vi "Update_Attribute_Tree_POLARIS.vi"(4 "Flush Tree?":bool, 5 "error in":errorcluster, 6 "Filter":string, 7 "Tree Control In":refnum<vi>, 8 "Camera Name In":T1 caption="Session In") -> (0 "error out":errorcluster, 2 "Tree Control Out":refnum<vi>, 3 "Session Out":T1)   [LabVIEW 2014, in "Camera Settings Dialog.lvlib" / "Camera Settings Dialog.lvclass"]
doc: "The Update Attribute Tree subVI, enumerates the attributes available for the camera and populates the Attribute Tree control with the attribute list."
uses:
  Camera Settings Dialog.lvclass
  <vilib>/userdefined/High Color/IMAQdx.ctl
  <vilib>/vision/driver/NI_Vision_Acquisition_Software.lvlib
  <resource>/objmgr/imaqdx.rc
panel:
  out "ValuesArray":string[](array[string])
  out "AttibuteArray":string[](array[string])
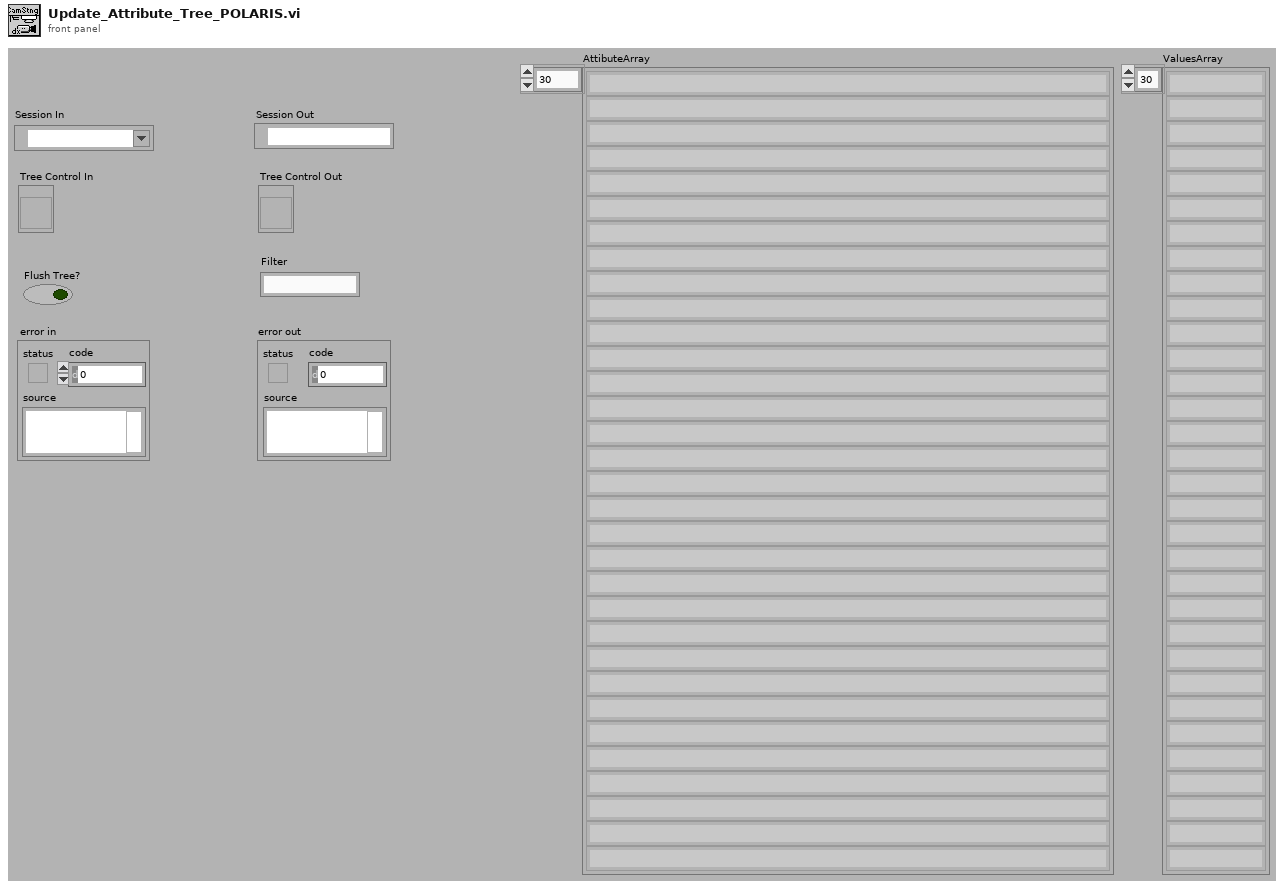
[diagram p1: front panel]
types:
  T1 = typedef "IMAQdx.ctl" = refnum<k21>
  T2 = typedef "NI_Vision_Acquisition_Software.lvlib/IMAQdx Attribute Type.ctl" = enum32{"U32", "I64", "DBL", "String", "Enum", "Bool", "Command"}
  T3 = cluster{"Attribute Type":T2, "Readable":bool, "Writable":bool, "Attribute Name":string}[]
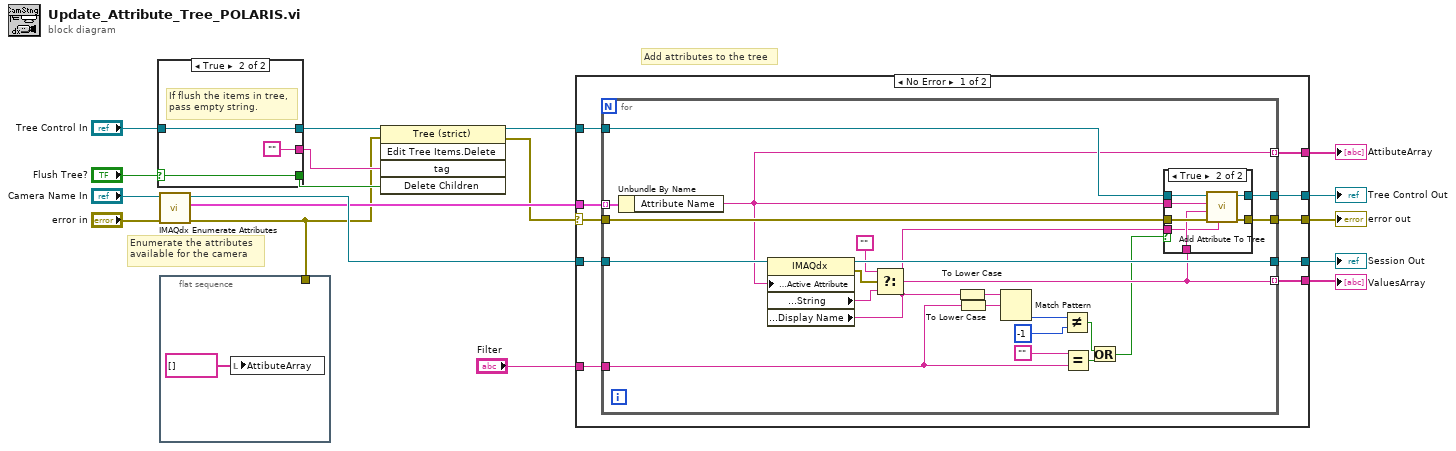
[diagram p0: block diagram]
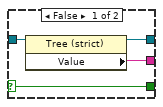
[diagram p2: hidden frame]
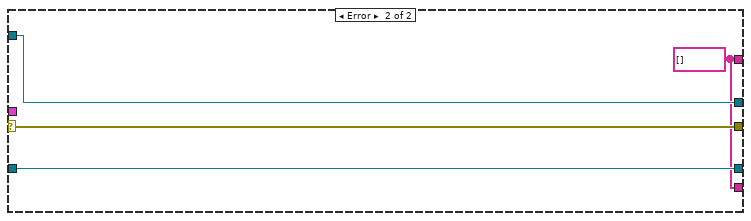
[diagram p4: hidden frame]
diagram:
  # "Add attributes to the tree"
  # "Enumerate the attributes \navailable for the camera"
  n1 = case shown="True" "Flush Tree?" {
    selector: "Flush Tree?" -> [w22 w25]
    tunnel: [w22 w25] -> w8
    tunnel: [w19 ""] -> w7
    tunnel: "Tree Control In" -> [w21 w23]
    tunnel: [w20 w23] -> w5
    frame False {
      n2 = property class="Tree (strict)"(reference=w21) -> (reference out=w20:refnum<vi>, "Value"=w19:string)  [unwired: 1 in, 1 out]
    }
    frame True {
      # "If flush the items in tree,\npass empty string."
    }
  }
  n3 = call <vilib>:"IMAQdx Enumerate Attributes.vi"("error in"="error in", "Session In"="Camera Name In") -> ("error out"=w3:errorcluster, "Attribute Information Array"=w17:T3, "Session Out"=w18:T1)  [unwired: 7 in]
  n4 = flat-sequence {
    tunnel: w3 -> [_]
    frame #0 {
      n5 = local write "AttibuteArray"(string[] []) -> ()
    }
  }
  n6 = invoke class="Tree (strict)" method="Edit Tree Items.Delete"(reference=w5, error in=w3, "tag"=w7, "Delete Children"=w8) -> (reference out=w12:refnum<vi>, error out=w11:errorcluster)  [unwired: 1 in, 3 out]
  n7 = case shown="No Error" w11 {
    selector: w11 -> [w34 w71]
    tunnel: w17 -> [w36 _]
    tunnel: w12 -> [w35 w69]
    tunnel: w18 -> [w33 w70]
    tunnel: [w32 w71] -> w10
    tunnel: [w31 w70] -> w14
    tunnel: [w30 w69] -> w13
    tunnel: [w29 w68] -> w4
    tunnel: [w28 w68] -> w2
    tunnel: "Filter" -> [w27 _]
    frame No Error {
      n8 = for {
        tunnel: w36 -> [w58] mode=indexing
        tunnel: w35 -> [w54]
        tunnel: w34 -> [w53]
        tunnel: w33 -> [w57]
        tunnel: [w56] -> w32
        tunnel: [w55] -> w31
        tunnel: [w52] -> w30
        tunnel: [w49] -> w29 mode=indexing
        tunnel: [w51] -> w28 mode=indexing
        tunnel: w27 -> [w48]
        n9 = Unbundle By Name(w58) -> ("Attribute Name"=w49:string)
        n10 = property class="IMAQdx"(reference=w57, "Camera Attributes:Active Attribute"=w49) -> (reference out=w55:T1, error out=w43:errorcluster, "Camera Attributes:Value:String"=w41:string, "Camera Attributes:Display Name"=w39:string)  [unwired: 1 in]
        n11 = Select(t="", s=w43, f=w41) -> (s? t:f=w51:string)
        n12 = To Lower Case(string=w39) -> (all lower case string=w38:string)
        n13 = To Lower Case(string=w48) -> (all lower case string=w37:string)
        n14 = Match Pattern(string=w38, regular expression=w37) -> (offset past match=w47:i32)  [unwired: 1 in, 3 out]
        n15 = Not Equal?(x=w47, y=-1) -> (x != y?=w44:bool)
        n16 = Equal?(x="", y=w48) -> (x = y?=w45:bool)
        n17 = Or(x=w44, y=w45) -> (x .or. y?=w40:bool)
        n18 = case shown="True" w40 {
          tunnel: [w59 w67] -> w56
          tunnel: w54 -> [w60 w66]
          tunnel: w53 -> [w59 w65]
          tunnel: [w60 w64] -> w52
          tunnel: w51 -> [_ w63]
          tunnel: w49 -> [_ w62]
          tunnel: w39 -> [_ w61]
          frame False {
          }
          frame True {
            n19 = call "Add Attribute To Tree.vi"("Display Name"=w61, "error in"=w65, "Value"=w63, "Attribute Name"=w62, "Attribute Table In"=w66) -> ("error out"=w67:errorcluster, "Attribute Table Out"=w64:refnum<vi>)  [unwired: 5 in]
          }
        }
      }
    }
    frame Error {
      w68 = string[] []
    }
  }
  "error out" <- w10
  "Session Out" <- w14
  "Tree Control Out" <- w13
  "AttibuteArray" <- w4
  "ValuesArray" <- w2
